vi "DAQmx Create Channel (AI-Force-Bridge-Table).vi"(0 "task in":refnum<k21>, 1 "maximum value":dbl=100.0 format="%0.2f", 2 "minimum value":dbl=-100.0 format="%0.2f", 3 "bridge information":T1={"bridge configuration"=10182, "voltage excitation source"=10200, "voltage excitation value"=2.5, "nominal bridge resistance"=350.0} {"voltage excitation source" items=["Internal"=10200, "External"=10167]; "bridge configuration" items=["Full Bridge"=10182, "Half Bridge"=10187, "Quarter Bridge"=10270]}, 5 "physical channels":tag, 7 "name to assign":string, 9 "units":i32(ring)=15876 items=["Newtons"=15875, "Pounds"=15876, "kgf"=15877, "From Custom Scale"=10065], 11 "error in":errorcluster, 12 "custom scale name":tag, 14 "scaling information":T2={"electrical values"=[-2.0, 0.0, 2.0], "electrical units"=15897, "physical values"=[-100.0, 0.0, 100.0], "physical units"=15876} {"physical units" items=["Newtons"=15875, "Pounds"=15876, "kgf"=15877]; "electrical units" items=["Volts/Volt"=15896, "mVolts/Volt"=15897]}) -> (4 "task out":refnum<k21>, 15 "error out":errorcluster)   [LabVIEW 2013]
doc: "Creates channel(s) that use a Wheatstone bridge to measure force or load. Use this instance with sensors whose specifications provide a table of electrical values and the corresponding physical values. When you use this scaling type, NI-DAQmx performs linear scaling between each pair of electrical and physical values. The input limits specified with <B>minimum value</B> and <B>maximum value</B> must fall within the smallest and largest physical values. For any data outside those endpoints, NI-DAQmx coerces that data to the endpoints."
uses:
  <resource>/objmgr/daqmx.rc
panel:
  # "input limits"
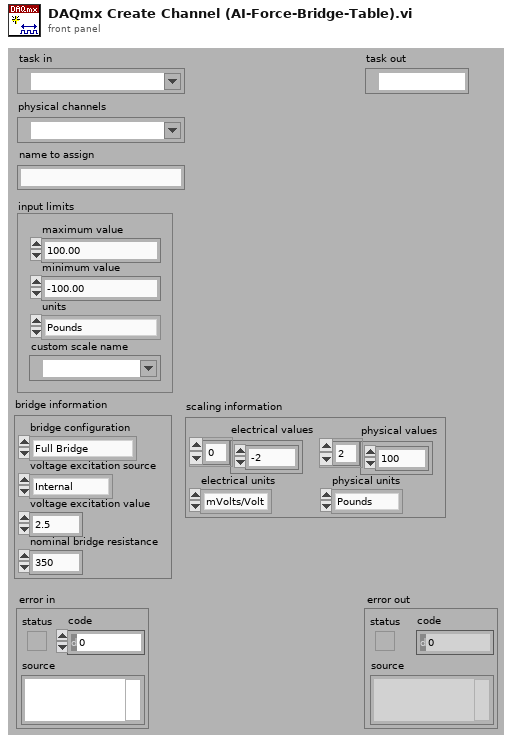
[diagram p1: front panel]
types:
  T1 = cluster{"bridge configuration":i32, "voltage excitation source":i32, "voltage excitation value":dbl, "nominal bridge resistance":dbl}
  T2 = cluster{"electrical values":dbl[], "electrical units":i32, "physical values":dbl[], "physical units":i32}
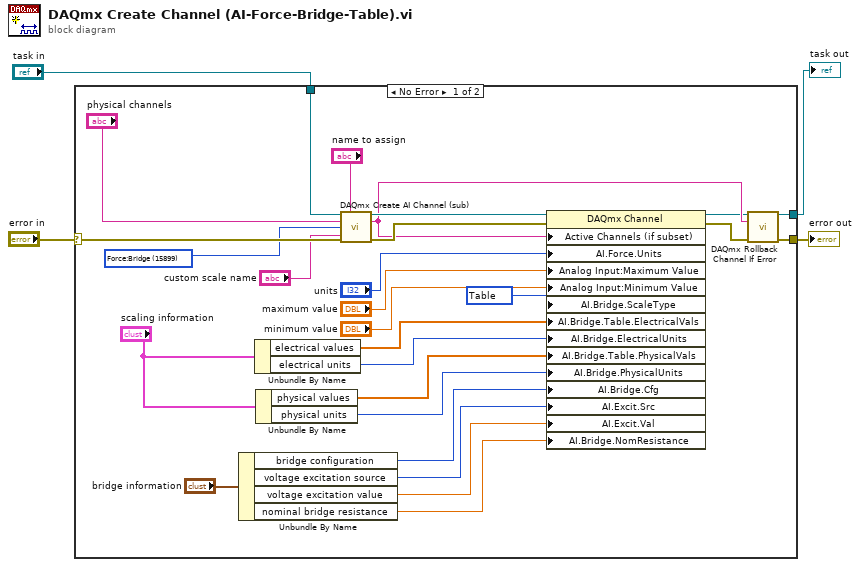
[diagram p0: block diagram]
diagram:
  n1 = case shown="No Error" "error in" {
    selector: "error in" -> [w30 w32]
    tunnel: [w22 w32] -> w4
    tunnel: "task in" -> [w31 w33]
    tunnel: [w21 w33] -> w1
    frame No Error {
      w5 = 15899 items=["Voltage"=10322, "Voltage RMS"=10350, "Current"=10134, "Current RMS"=10351, "More:Voltage:Custom with Excitation"=10323, "More:Bridge (V/V)"=15908, "Frequency"=10181, "Resistance"=10278, "Temperature:Thermocouple"=10303, "Temperature:Thermistor"=10302, "Temperature:RTD"=10301, "Temperature:Built-in Sensor"=10311, "Strain Gage"=10300, "Position:LVDT"=10352, "Position:RVDT"=10353, "Position:Eddy Current Proximity Probe"=14835, "Accelerometer"=10356, "Force:Bridge"=15899, "Force:IEPE Sensor"=15895, "Pressure:Bridge"=15902, "Sound Pressure:Microphone"=10354, "Torque:Bridge"=15905, "TEDS Sensor"=12531] ("AI.MeasType")
      w7 = 10450 items=["None"=10230, "Two-Point Linear"=15898, "Table"=10450, "Polynomial"=10449] ("AI.Bridge.ScaleType")
      n2 = Unbundle By Name("bridge information") -> ("bridge configuration"=w11:i32, "voltage excitation source"=w10:i32, "voltage excitation value"=w9:dbl, "nominal bridge resistance"=w8:dbl)
      n3 = Unbundle By Name("scaling information") -> ("electrical values"=w16:dbl[], "electrical units"=w15:i32)
      n4 = Unbundle By Name("scaling information") -> ("physical values"=w14:dbl[], "physical units"=w13:i32)
      n5 = call "DAQmx Create AI Channel (sub).vi"("task in"=w31, "virtual channel name"="name to assign", "physical channel name"="physical channels", "measurement type"=w5, "error in"=w30, "custom scale"="custom scale name") -> ("task out"=w23:refnum<k21>, "channel names"=w20:string, "error out"=w28:errorcluster)  [unwired: 7 out]
      n6 = property class="DAQmx Channel"(reference=w23, error in=w28, "Active Channels (if subset)"=w20, "AI.Force.Units"="units", "Analog Input:Maximum Value"="maximum value", "Analog Input:Minimum Value"="minimum value", "AI.Bridge.ScaleType"=w7, "AI.Bridge.Table.ElectricalVals"=w16, "AI.Bridge.ElectricalUnits"=w15, "AI.Bridge.Table.PhysicalVals"=w14, "AI.Bridge.PhysicalUnits"=w13, "AI.Bridge.Cfg"=w11, "AI.Excit.Src"=w10, "AI.Excit.Val"=w9, "AI.Bridge.NomResistance"=w8) -> (reference out=w18:refnum<k21>, error out=w17:errorcluster)
      n7 = call "DAQmx Rollback Channel If Error.vi"("task in"=w18, "channel names"=w20, "error in"=w17) -> ("task out"=w21:refnum<k21>, "error out"=w22:errorcluster)  [unwired: 11 out]
    }
    frame Error {
    }
  }
  "error out" <- w4
  "task out" <- w1
